vi "Write Value (Signaling).vi"(8 "error in (no error)":errorcluster, 10 "Value (Signaling)":variant, 11 "DoValueSignal in":refnum<class "DoValueSignal.lvclass">) -> (0 "error out":errorcluster, 3 "DoValueSignal out":refnum<class "DoValueSignal.lvclass">)   [LabVIEW 2016, in "DoValueSignal.lvclass"]
uses:
  DoValueSignal.lvclass
  DoValueSignal.lvclass/DoValueSignal.ctl
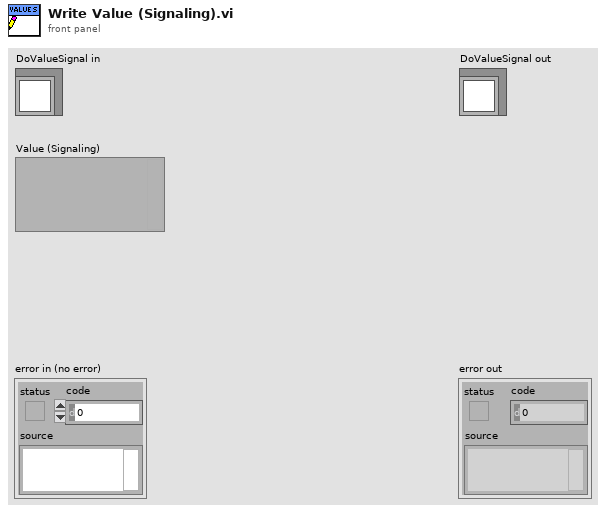
[diagram p1: front panel]
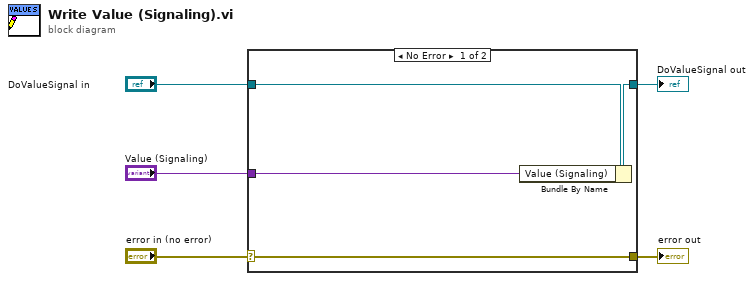
[diagram p0: block diagram]
diagram:
  n1 = case shown="No Error" "error in (no error)" {
    selector: "error in (no error)" -> [w9 w10]
    tunnel: [w9 w10] -> w4
    tunnel: [w7 w11] -> w2
    tunnel: "DoValueSignal in" -> [w8 w11]
    tunnel: "Value (Signaling)" -> [w6 _]
    frame No Error {
      n2 = Bundle By Name(cluster=w8, "Value (Signaling)"=w6) -> (w7:refnum<class "DoValueSignal.lvclass">)
    }
    frame Error {
    }
  }
  "error out" <- w4
  "DoValueSignal out" <- w2
